vi "Condition Msg Output IMO VI.vi"(6 "Name":string, 8 "error in":errorcluster, 9 "Msg Output All Terminals (For Init Msg Output.vi)":i32[](array[numeric]), 10 "Name Msg Output Refs.Init Msg Output VI":refnum<vi>) -> (0 "error out":errorcluster)   [LabVIEW 2025, in "_Rescript.lvlib" / "Msg.lvlib" / "Msg.lvclass"]
uses:
  <vilib>/Utility/traverseref.llb/TRef TravTarget.ctl
  Msg.lvclass
  Msg.lvclass/Msg.ctl
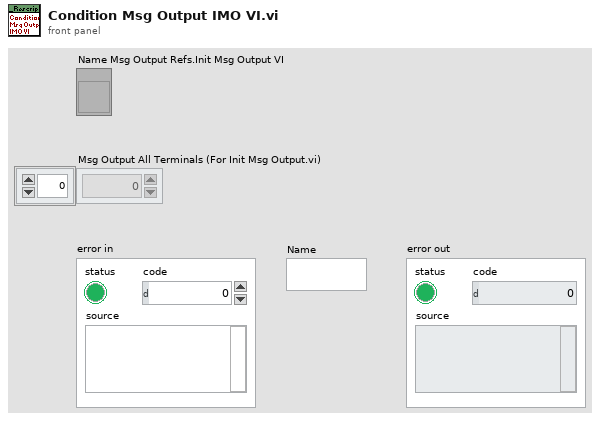
[diagram p1: front panel]
types:
  T1 = typedef "TRef TravTarget.ctl" = enum16{"FP", "BD", "Other"}
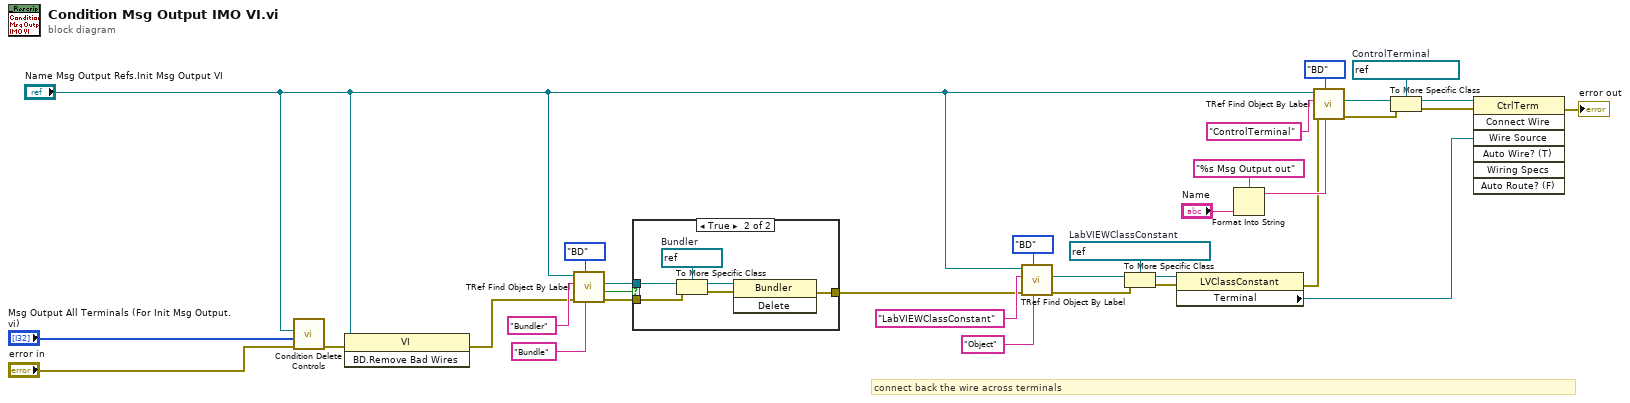
[diagram p0: block diagram]
diagram:
  w18 = refnum<vi> refnum  # ControlTerminal
  w30 = refnum<vi> refnum  # LabVIEWClassConstant
  # "connect back the wire across terminals"
  n1 = call "Condition Delete Controls.vi"("error in"="error in", "Terminals"="Msg Output All Terminals (For Init Msg Output.vi)", "VI"="Name Msg Output Refs.Init Msg Output VI") -> ("error out"=w7:errorcluster)  [unwired: 8 in]
  n2 = invoke class="VI" method="BD.Remove Bad Wires"(reference="Name Msg Output Refs.Init Msg Output VI", error in=w7) -> (error out=w6:errorcluster)  [unwired: 1 in, 2 out]
  n3 = call <vilib>:"TRef Find Object By Label.vi"("Label"="Bundle", "Traverse Target"=TRef_TravTarget."BD", "error in (no error)"=w6, "Class Name"="Bundler", "VI Ref"="Name Msg Output Refs.Init Msg Output VI") -> ("error out"=w12:errorcluster, "Found?"=w5:bool, "Found Obj Ref"=w11:refnum<vi>)  [unwired: 3 in, 1 out]
  n4 = case shown="True" w5 {
    tunnel: w12 -> [w34 w40]
    tunnel: w11 -> [_ w38]
    tunnel: [w34 w35] -> w4
    frame False {
    }
    frame True {
      w39 = refnum<vi> refnum  # Bundler
      n5 = To More Specific Class(target class=w39, reference=w38, error in=w40) -> (specific class reference=w37:refnum<vi>, error out=w36:errorcluster)
      n6 = invoke class="Bundler" method="Delete"(reference=w37, error in=w36) -> (error out=w35:errorcluster)  [unwired: 1 in, 2 out]
    }
  }
  n7 = call <vilib>:"TRef Find Object By Label.vi"("Label"="Object", "Traverse Target"=TRef_TravTarget."BD", "error in (no error)"=w4, "Class Name"="LabVIEWClassConstant", "VI Ref"="Name Msg Output Refs.Init Msg Output VI") -> ("error out"=w31:errorcluster, "Found Obj Ref"=w29:refnum<vi>)  [unwired: 3 in, 2 out]
  n8 = To More Specific Class(target class=w30, reference=w29, error in=w31) -> (specific class reference=w26:refnum<vi>, error out=w24:errorcluster)
  n9 = property class="LVClassConstant"(reference=w26, error in=w24) -> (error out=w15:errorcluster, "Terminal"=w13:refnum<vi>)  [unwired: 1 out]
  n10 = Format Into String(format string="%s Msg Output out", "Name") -> (resulting string=w21:string)  [unwired: 2 in, 1 out]
  n11 = call <vilib>:"TRef Find Object By Label.vi"("Label"=w21, "Traverse Target"=TRef_TravTarget."BD", "error in (no error)"=w15, "Class Name"="ControlTerminal", "VI Ref"="Name Msg Output Refs.Init Msg Output VI") -> ("error out"=w19:errorcluster, "Found Obj Ref"=w20:refnum<vi>)  [unwired: 3 in, 2 out]
  n12 = To More Specific Class(target class=w18, reference=w20, error in=w19) -> (specific class reference=w16:refnum<vi>, error out=w14:errorcluster)
  n13 = invoke class="CtrlTerm" method="Connect Wire"(reference=w16, error in=w14, "Wire Source"=w13) -> (error out=→"error out":errorcluster)  [unwired: 4 in, 6 out]
